vi "SetTemperature.vi"() -> ()   [LabVIEW 2013]
panel:
  in  "error in (no error)":errorcluster
  in  "Set Temperature (K)":dbl
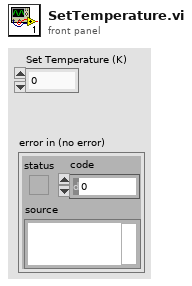
[diagram p1: front panel]
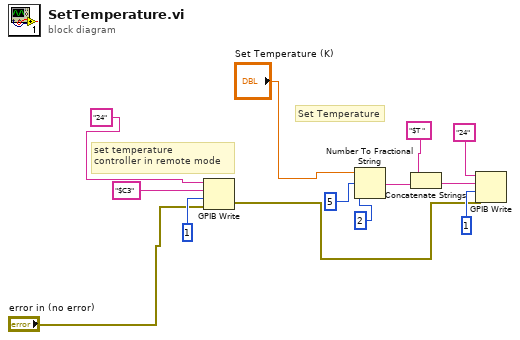
[diagram p0: block diagram]
diagram:
  # "set temperature\ncontroller in remote mode"
  # "Set Temperature"
  n1 = GPIB Write(0:"24", 1:"$C3", 2:1, 3:"error in (no error)") -> (6:w2:errorcluster)  [unwired: 1 in, 1 out]
  n2 = Number To Fractional String(number="Set Temperature (K)", width (-)=5, precision (6)=2) -> (F-format string=w11:string)  [unwired: 1 in]
  n3 = Concatenate Strings("$T ", w11) -> (w10:string)
  n4 = GPIB Write(0:"24", 1:w10, 2:1, 3:w2) -> ()  [unwired: 1 in, 2 out]
